vi "Quaternion_Get_All.vi"(11 "Quaternion":T1={"R"=1.0, "V"=[0.0, 0.0, 0.0]}) -> (0 "Z":dbl, 1 "Y":dbl, 2 "X":dbl, 3 "W":dbl=1.0)   [LabVIEW 2019, in "Trajectory_Library.lvlib"]
doc: "Return the W, X, Y, and Z components of the quaternion\n\nParameters:\n - Quaternion -- The quaternion data cluster. \n\nReturns:\n - W - Returns W component of the quaternion.\n - X - Returns X component of the quaternion.\n - Y - Returns Y component of the quaternion.\n - Z - Returns Z component of the quaternion."
uses:
  TypeDef/QUATERNION.ctl
  Trajectory_Library.lvlib
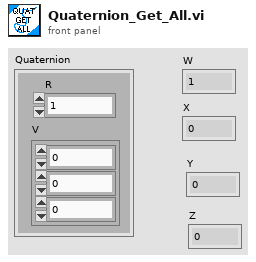
[diagram p1: front panel]
types:
  T1 = typedef "Trajectory_Library.lvlib/QUATERNION.ctl" = cluster{"R":dbl, "V":dbl[]}
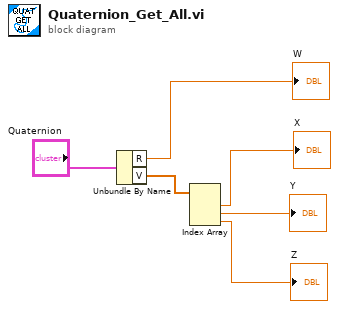
[diagram p0: block diagram]
diagram:
  n1 = Unbundle By Name("Quaternion") -> ("R"=→"W":dbl, "V"=w4:dbl[])
  n2 = Index Array(array=w4) -> (element #1=→"X":dbl, element #2=→"Y":dbl, element #3=→"Z":dbl)  [unwired: 3 in]
